vi "Error_Log.vi"(8 "error in":errorcluster, 10 "Level of the Error":string(combo), 11 "Error report":errorcluster) -> (0 "error out":errorcluster)   [LabVIEW 2020]
doc: "Writte Log in TXT file"
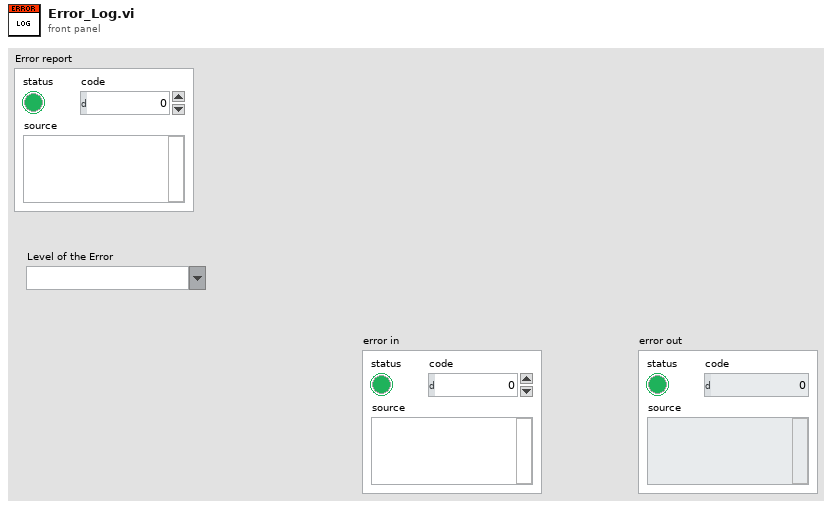
[diagram p1: front panel]
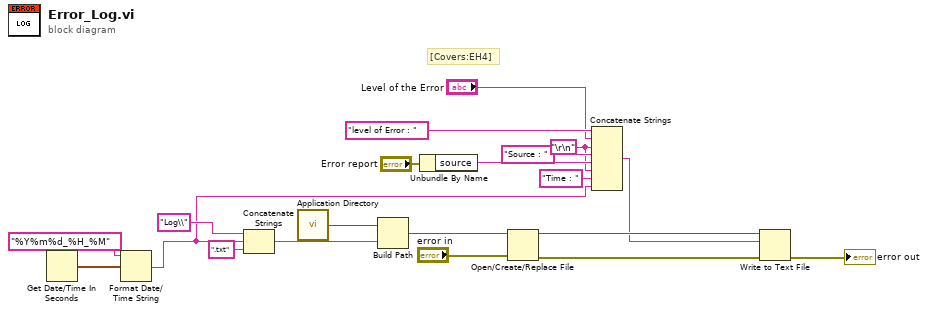
[diagram p0: block diagram]
diagram:
  w5 = "\r\n"
  # "[Covers:EH4]"
  n1 = Get Date/Time In Seconds() -> (seconds since 1Jan1904=w3:timestamp)
  n2 = Format Date/Time String(time format string (%c)="%Y%m%d_%H_%M", seconds (now)=w3) -> (date/time string=w1:string)  [unwired: 1 in]
  n3 = Concatenate Strings("Log\\", w1, ".txt" ("string")) -> (w18:string)
  n4 = call <vilib>:"Application Directory.vi"() -> ("Application Directory"=w20:path)
  n5 = Build Path(base path=w20, name or relative path=w18) -> (appended path=w14:path)
  n6 = Unbundle By Name("Error report") -> ("source"=w10:string)
  n7 = Open/Create/Replace File(file path (use dialog)=w14, error in="error in") -> (refnum out=w13:refnum<file>, error out=w11:errorcluster)  [unwired: 4 in, 1 out]
  n8 = Concatenate Strings("level of Error : " ("string"), "Level of the Error", w5, "Source : " ("string"), w10, w5, "Time : " ("string"), w1) -> (w8:string)
  n9 = Write to Text File(file (use dialog)=w13, text=w8, error in=w11) -> (error out=→"error out":errorcluster)  [unwired: 1 in, 2 out]
